vi "CurrentMonitoring.vi"() -> ()   [LabVIEW 2018]
panel:
  in  "Elevator_1_PDP":i8
  in  "Elevator_2_PDP":i8
  in  "Elevator_3_PDP":i8
  in  "Lower_Intake_PDP":i8
  in  "Elevator_4_PDP":i8
  in  "Upper_Intake_PDP":i8
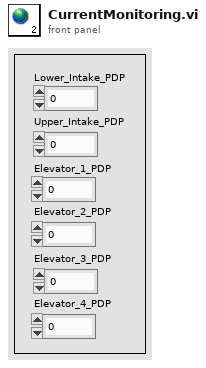
[diagram p1: front panel]
diagram:
